vi "Create.vi"() -> (3 "Recipe State Data":refnum<data-value>)   [LabVIEW 2022 SP3, in "Recipe State Data.lvclass"]
uses:
  Recipe State Data.lvclass
  Recipe State Data.lvclass/Recipe State Data.ctl
panel:
  in  "Current Recipe Iterations":dbl
  in  "Desired Recipe Iterations":dbl
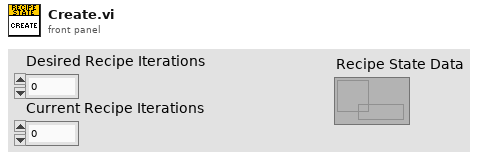
[diagram p1: front panel]
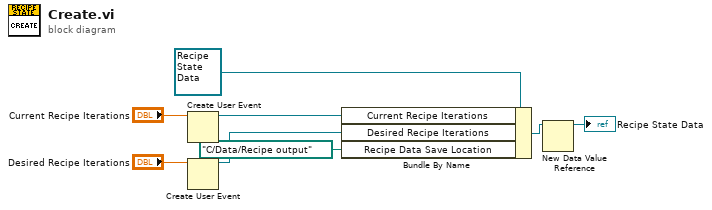
[diagram p0: block diagram]
diagram:
  n1 = Create User Event(user event datatype="Current Recipe Iterations") -> (user event=w3:refnum<user-event>)  [unwired: 1 in, 1 out]
  n2 = Create User Event(user event datatype="Desired Recipe Iterations") -> (user event=w2:refnum<user-event>)  [unwired: 1 in, 1 out]
  n3 = Bundle By Name(cluster=refnum<class "Recipe State Data.lvclass"> refnum ("Recipe State Data in"), "Current Recipe Iterations"=w3, "Desired Recipe Iterations"=w2, "Recipe Data Save Location"=path "C:/Data/Recipe output") -> (w7:refnum<class "Recipe State Data.lvclass">)
  n4 = New Data Value Reference(data value=w7) -> (data value reference=→"Recipe State Data":refnum<data-value>)  [unwired: 1 in, 1 out]
